vi "acquisitionStart.vi"(6 "Delay between send and receive [ms]":i32=100, 8 "error in (no error)":errorcluster, 10 "openShutter":bool=TRUE, 11 "CCD in":refnum<class "CCD.lvclass">) -> (0 "error out":errorcluster, 1 "ID":i32, 2 "results-JSON string":string, 3 "CCD out":refnum<class "CCD.lvclass">)   [LabVIEW 2023, in "horiba.lvlib" / "CCD.lvclass"]
doc: "tarts an acquisition that has been set up according to the previously defined acquisition parameters.\n\nNote: To specify the acquisition parameters please see ccd_setROI and ccd_setXAxisConversionType. If there are no acquisition parameters specified at the time of acquisition it may result in no data being generated."
uses:
  CCD.lvclass
  20f7d3bd-08ac-4524-9bed-df36c1da25a0.vi
  cab240a6-cbf4-4e2c-ab79-96d9c1b88265.vi
  <vilib>/JDP Science/JSONtext/Variant to JSON Text.vi
  <vilib>/JDP Science/JSONtext/Set Item.vi
  <vilib>/JDP Science/JSONtext/LVClass Serializer/JSONtext LVClass Serializer.lvclass
  GenericDevice/GenericDevice.lvclass
  <vilib>/JDP Science/JSONtext/JSONtext.lvlib
panel:
  # "Connector Pane"
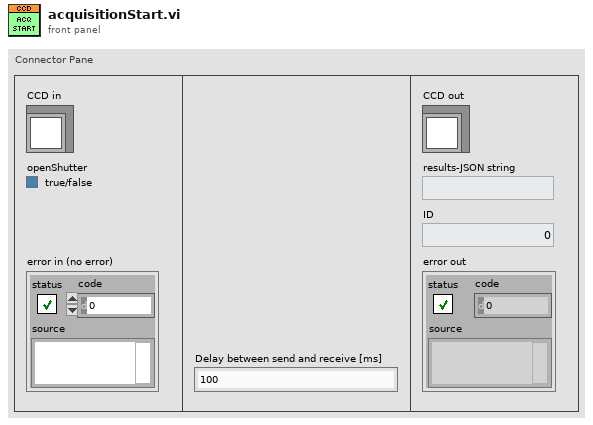
[diagram p1: front panel]
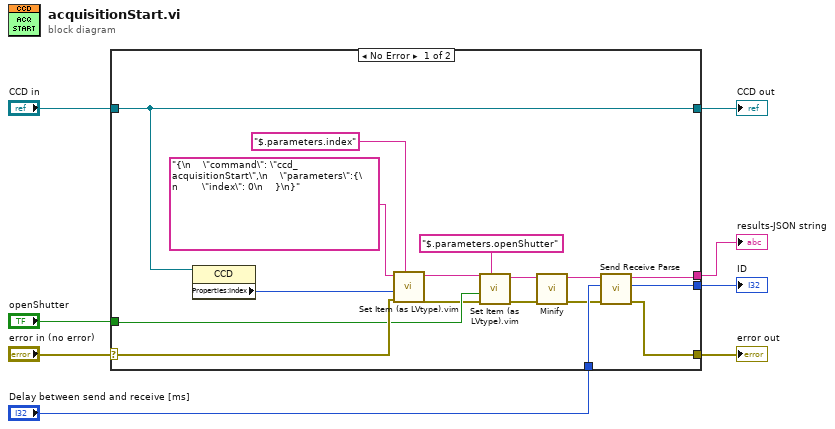
[diagram p0: block diagram]
diagram:
  n1 = case shown="No Error" "error in (no error)" {
    selector: "error in (no error)" -> [w21 w27]
    tunnel: [w16 w27] -> w7
    tunnel: [w23 w26] -> w5
    tunnel: "CCD in" -> [w23 w26]
    tunnel: "openShutter" -> [w19 _]
    tunnel: [w15 _] -> w4
    tunnel: [w14 _] -> w3
    tunnel: "Delay between send and receive [ms]" -> [w12 _]
    frame No Error {
      n2 = property class="CCD"(reference=w23) -> ("Properties:Index"=w22:i32)  [unwired: 1 in, 2 out]
      n3 = call "Set Item (as LVtype).vim"("$Path or Item Name"="$.parameters.index", "error in (no error)"=w21, "Anything"=w22, "JSON"="{\n    \"command\": \"ccd_acquisitionStart\",\n    \"parameters\":{\n        \"index\": 0\n    }\n}") -> ("error out"=w18:errorcluster, "<JSON>"=w17:string)  [unwired: 4 in, 1 out]
      n4 = call "Set Item (as LVtype).vim"("$Path or Item Name"="$.parameters.openShutter", "error in (no error)"=w18, "Anything"=w19, "JSON"=w17) -> ("error out"=w11:errorcluster, "<JSON>"=w13:string)  [unwired: 4 in, 1 out]
      n5 = call <vilib>:"Minify.vi"("error in (no error)"=w11, "JSON"=w13) -> ("error out"=w10:errorcluster, "<JSON>"=w9:string)  [unwired: 7 in, 1 out]
      n6 = call "Send Receive Parse.vi"("error in"=w10, "Delay between send and receive [ms]"=w12, "<JSON>"=w9) -> ("error out"=w16:errorcluster, "ID"=w14:i32, "results-JSON string"=w15:string)  [unwired: 6 in]
    }
    frame Error {
    }
  }
  "error out" <- w7
  "CCD out" <- w5
  "results-JSON string" <- w4
  "ID" <- w3
